vi "Main Abstraction Level 4.vi"() -> ()   [LabVIEW 2019]
doc: "This is one of the levels of abstract design along the timeline leading to the goal of a complete measurement application."
uses:
  messages/MeasureAndLogMessage.lvclass/MeasureAndLogMessage.ctl
  subVIs/Measure and Log Settings.ctl
  subVIs/Simulated Signal Type.ctl
  <extravilib>/ChannelInstances/Stream-str/Read With Abort.vi
  <extravilib>/ChannelInstances/Lossy Stream-a[.](wfm(dbl))/Read With Abort.vi
  <resource>/Channels/Messenger/Read With Abort.vi
  <vilib>/ChannelSupport/Channel Message/Read ID.vi
  <extravilib>/ChannelInstances/Stream-a[.](wfm(dbl))/Endpoint.vi
  <extravilib>/ChannelInstances/Stream-str/EndpointRead.vi
  <extravilib>/ChannelInstances/Lossy Stream-a[.](wfm(dbl))/EndpointRead.vi
  <extravilib>/ChannelInstances/Lossy Stream-a[.](wfm(dbl))/Endpoint.vi
  <extravilib>/ChannelInstances/Stream-str/Endpoint.vi
  messages/MeasureAndLogMessage.lvclass
  e:/builds/penguin/labview/branches/2019/dev/dist/vi.lib/ChannelSupport/Channel Message/Channel Message.lvclass
  <extravilib>/ChannelInstances/Tag-path/Instantiate.vi
  <extravilib>/ChannelInstances/Stream-a[.](wfm(dbl))/Instantiate.vi
  <extravilib>/ChannelInstances/Lossy Stream-a[.](wfm(dbl))/Instantiate.vi
  <extravilib>/ChannelInstances/Lossy Stream-a[.](wfm(dbl))/)Channel.vi
  <resource>/ChannelSupport/_ChannelSupport/WaitIfNeeded.vi
  <extravilib>/ChannelInstances/Stream-str/Instantiate.vi
  <extravilib>/ChannelInstances/Stream-str/)Channel.vi
  <resource>/Channels/Messenger/Instantiate.vi
  <resource>/Channels/Messenger/Endpoint.vi
  <extravilib>/ChannelInstances/Tag-path/Endpoint.vi
  <extravilib>/ChannelInstances/Stream-a[.](wfm(dbl))/)Channel.vi
  <resource>/Channels/Messenger/Messenger.lvlib
  <extravilib>/ChannelInstances/Stream-str.lvlib
  <extravilib>/ChannelInstances/Lossy Stream-a[.](wfm(dbl)).lvlib
  <extravilib>/ChannelInstances/Tag-path.lvlib
  <extravilib>/ChannelInstances/Stream-a[.](wfm(dbl)).lvlib
panel:
  in  "Exit flag":bool
  in  "Record":bool
  in  "Stop":bool
  out "Data":waveform(dbl)[](graph)
  out "Status":string
  in  "Settings":bool
  in  "Start":bool
  in  "Exit":bool
  # "Continuous Measurement Data Logger"
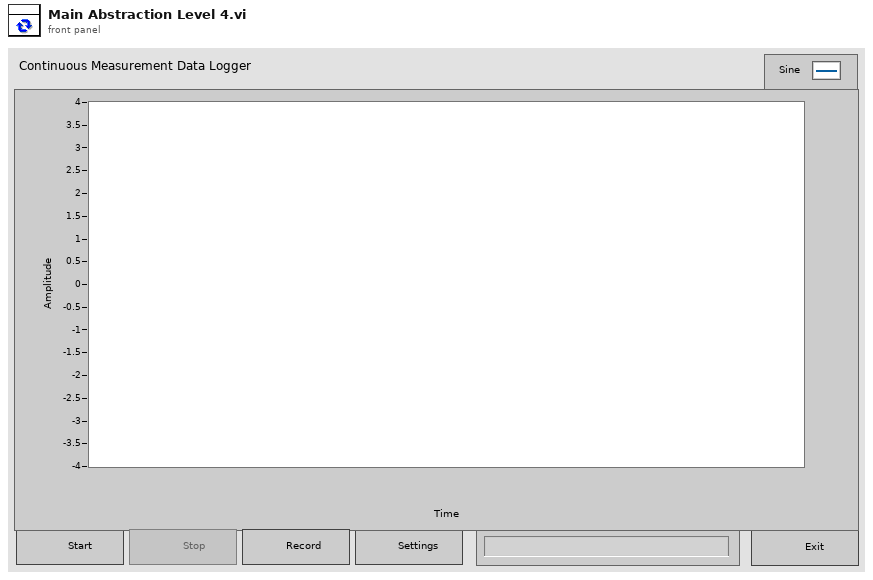
[diagram p1: front panel]
types:
  T1 = typedef "Measure and Log Settings.ctl" = cluster{"sample rate":dbl, "input range":dbl, "logfile path":path, "Simulated Signal":cluster{"signal type":T2, "frequency":dbl, "amplitude":dbl}}
  T2 = typedef "Simulated Signal Type.ctl" = enum16{"Sine Wave", "Square Wave with Noise"}
  T3 = enum8{"Enabled", "Disabled", "Disabled and Grayed Out"}
  T4 = typedef "Messenger.lvlib/))Channel.ctl" = refnum<queue>
  T5 = typedef "Tag-path.lvlib/))Channel.ctl" = refnum<queue>
  T6 = typedef "Stream-a[.](wfm(dbl)).lvlib/)Channel.ctl" = refnum<queue>
  T7 = typedef "Stream-str.lvlib/)Channel.ctl" = refnum<queue>
  T8 = typedef "Lossy Stream-a[.](wfm(dbl)).lvlib/)Channel.ctl" = refnum<queue>
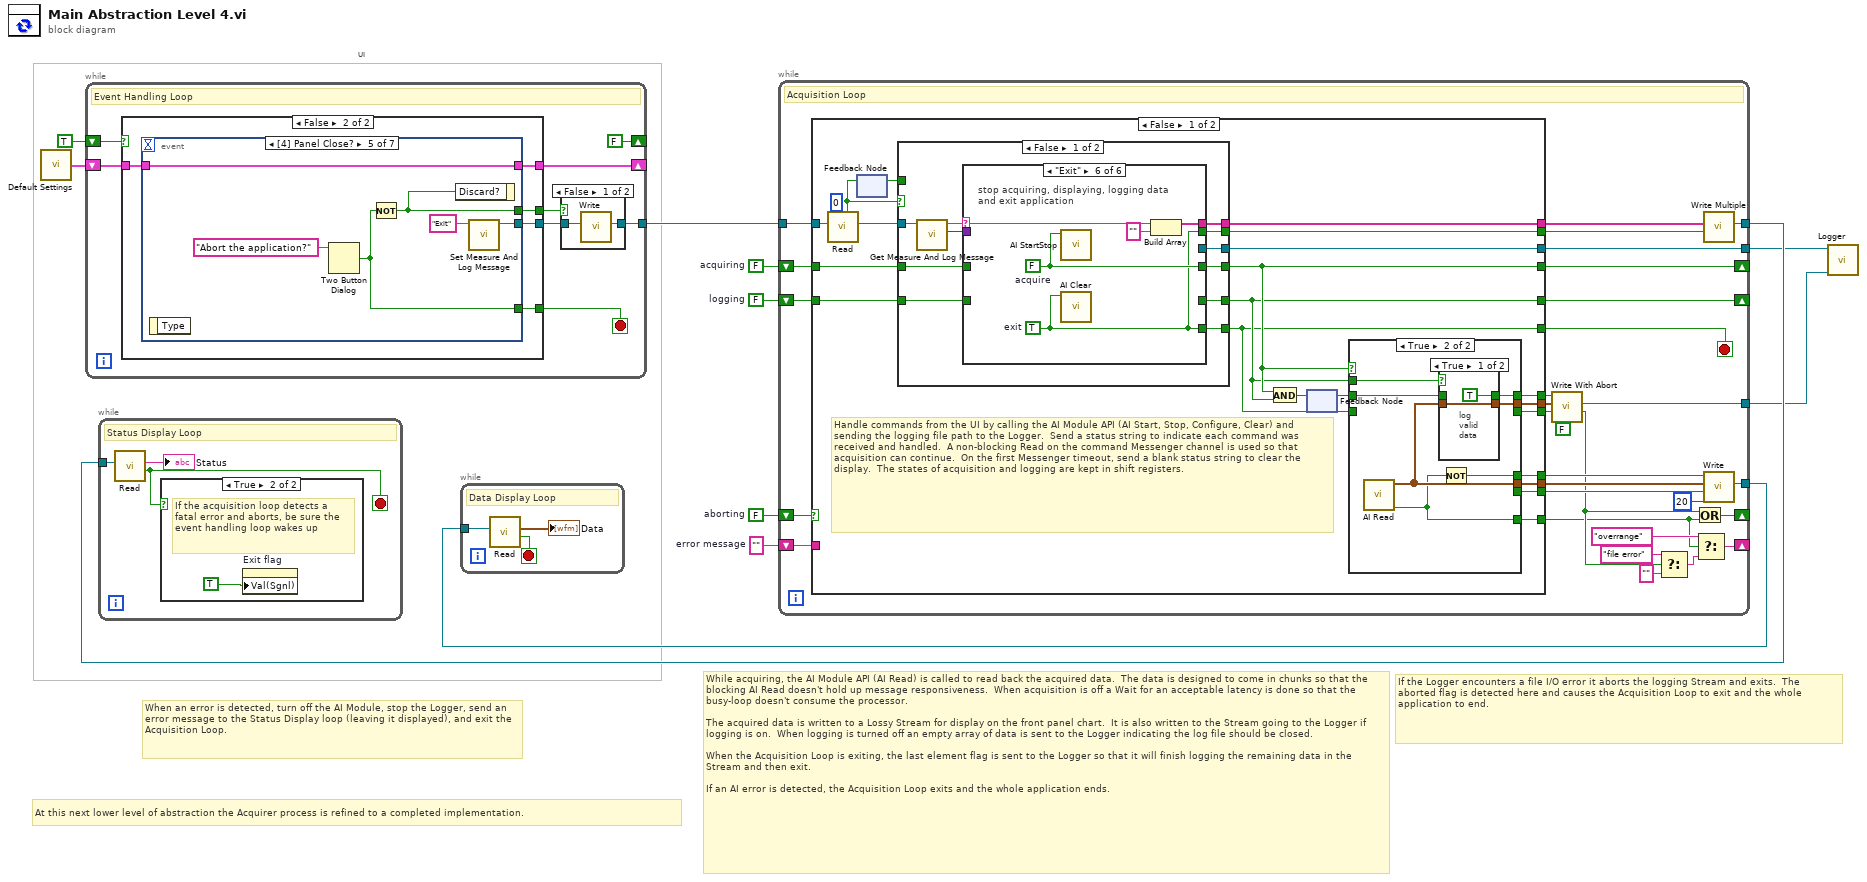
[diagram p0: block diagram]
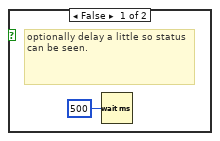
[diagram p2: hidden frame]
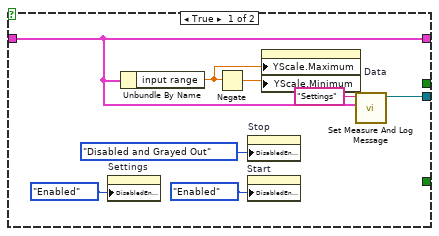
[diagram p3: hidden frame]
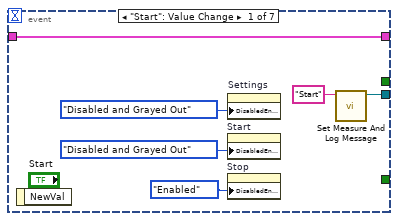
[diagram p4: hidden frame]
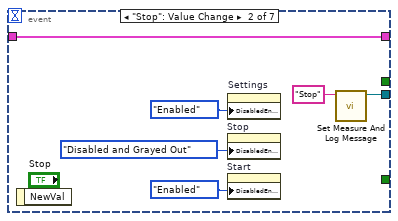
[diagram p5: hidden frame]
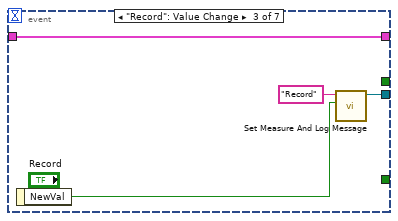
[diagram p6: hidden frame]
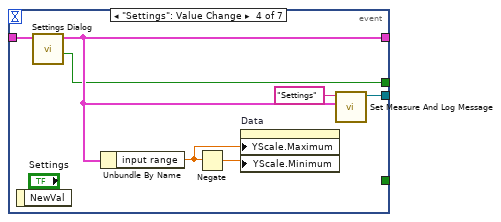
[diagram p7: hidden frame]
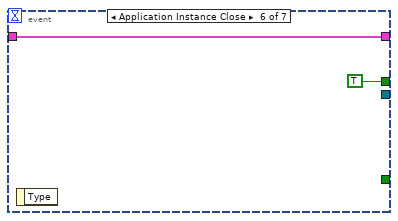
[diagram p8: hidden frame]
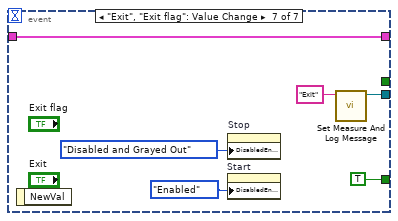
[diagram p9: hidden frame]
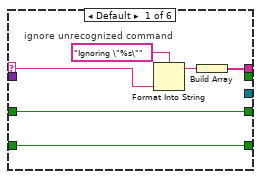
[diagram p11: hidden frame]
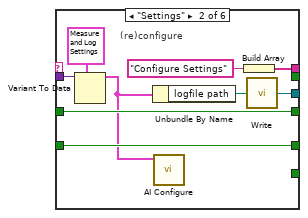
[diagram p12: hidden frame]
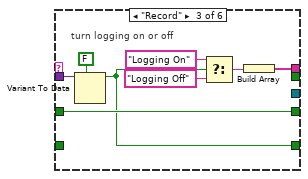
[diagram p13: hidden frame]
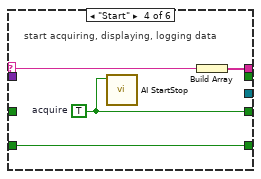
[diagram p14: hidden frame]
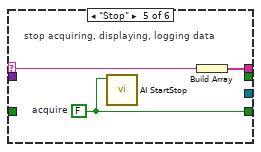
[diagram p15: hidden frame]
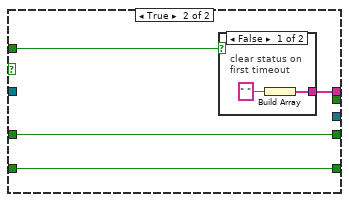
[diagram p16: hidden frame]
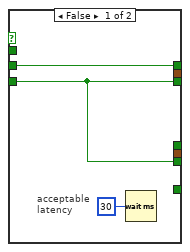
[diagram p18: hidden frame]
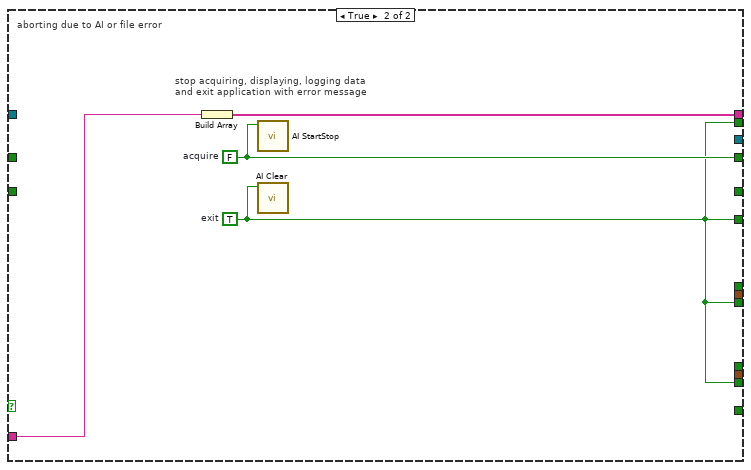
[diagram p20: hidden frame]
diagram:
  w6 = ""  # error message
  w8 = FALSE  # aborting
  w9 = FALSE  # logging
  w10 = FALSE  # acquiring
  # "At this next lower level of abstraction the Acquirer process is refined to a completed implementation."
  # "When an error is detected, turn off the AI Module, stop the Logger, send an error message to the Status Display loop (leaving it displayed), and exit the Acquisition Loop."
  # "If the Logger encounters a file I/O error it aborts the logging Stream and exits.  The aborted flag is detected here and causes the Acquisition Loop to exit and the whole application to end."
  # "While acquiring, the AI Module API (AI Read) is called to read back the acquired data.  The data is designed to come in chunks so that the blocking AI Read doesn't hold up message responsiveness.  When acquisition is off a Wait for an acceptable latency is done so that the busy-loop doesn't consume the processor.\n\nThe acquired data is written to a Lossy Stream for display on the front panel chart.  It is also written to the Stream going to the Logger if logging is on.  When logging is turned off an empty array of data is sent to the Logger indicating the log file should be closed.\n\nWhen the Acquisition Loop is exiting, the last element flag is sent to the Logger so that it will finish logging the remaining data in the Stream and then exit.\n\nIf an AI error is detected, the Acquisition Loop exits and the whole application ends."
  # "UI"
  n1 = call "Default Settings.vi"() -> ("default settings"=w7:T1)
  n2 = while {
    tunnel: [w16] -> w11
    shift-right: [w18] -> _
    shift-left: w7 -> [w17]
    shift-right: [FALSE] -> _
    shift-left: TRUE -> [w12]
    stop <- w19 stop-if-true
    # "Event Handling Loop"
    n3 = case shown="False" w12 {
      tunnel: [_ w32] -> w19
      tunnel: [w26 w31] -> w18
      tunnel: w17 -> [w26 w30]
      tunnel: [w22 w29] -> w15
      tunnel: [_ w28] -> w14
      frame True {
        n4 = property on="Settings" class="Bool"("DisabledEnum"=T3."Enabled" ("Disabled")) -> ()  [unwired: 2 in, 2 out]
        n5 = Unbundle By Name(w26) -> ("input range"=w20:dbl)
        n6 = Negate(x=w20) -> (-x=w21:dbl)
        n7 = property on="Stop" class="Bool"("DisabledEnum"=T3."Disabled and Grayed Out" ("Disabled")) -> ()  [unwired: 2 in, 2 out]
        n8 = property on="Start" class="Bool"("DisabledEnum"=T3."Enabled" ("Disabled")) -> ()  [unwired: 2 in, 2 out]
        n9 = property on="Data" class="WFChart (strict)"("YScale.Maximum"=w20, "YScale.Minimum"=w21) -> ()  [unwired: 2 in, 2 out]
        n10 = call "Set Measure And Log Message.vi"("args"=w26, "command"="Settings") -> ("MyMessage"=w22:refnum<class "MeasureAndLogMessage.lvclass">)  [unwired: 9 in]
      }
      frame False {
        n11 = event shown="[4] Panel Close?" {
          selector: _ -> [_ _ _ _ _ _ _]
          dyn-events: _ -> [_ _ _ _ _ _ _]
          timeout: _ -> [_ _ _ _ _ _ _]
          tunnel: [_ _ _ _ w57 _ TRUE] -> w32
          tunnel: [w34 w40 w46 w54 w60 w63 w65] -> w31
          tunnel: w30 -> [w34 w40 w46 w55 w60 w63 w65]
          tunnel: [w33 w39 w45 w53 w58 _ w64] -> w29
          tunnel: [_ _ _ w51 w56 TRUE ("cancelled") _] -> w28
          event "Start": Value Change {
            n12 = event-data() -> ()  [unwired: 1 in, 1 out]
            n13 = property on="Settings" class="Bool"("DisabledEnum"=T3."Disabled and Grayed Out" ("Disabled")) -> ()  [unwired: 2 in, 2 out]
            n14 = property on="Start" class="Bool"("DisabledEnum"=T3."Disabled and Grayed Out" ("Disabled")) -> ()  [unwired: 2 in, 2 out]
            n15 = property on="Stop" class="Bool"("DisabledEnum"=T3."Enabled" ("Disabled")) -> ()  [unwired: 2 in, 2 out]
            n16 = call "Set Measure And Log Message.vi"("command"="Start") -> ("MyMessage"=w33:refnum<class "MeasureAndLogMessage.lvclass">)  [unwired: 10 in]
          }
          event "Stop": Value Change {
            n17 = event-data() -> ()  [unwired: 1 in, 1 out]
            n18 = property on="Settings" class="Bool"("DisabledEnum"=T3."Enabled" ("Disabled")) -> ()  [unwired: 2 in, 2 out]
            n19 = property on="Stop" class="Bool"("DisabledEnum"=T3."Disabled and Grayed Out" ("Disabled")) -> ()  [unwired: 2 in, 2 out]
            n20 = property on="Start" class="Bool"("DisabledEnum"=T3."Enabled" ("Disabled")) -> ()  [unwired: 2 in, 2 out]
            n21 = call "Set Measure And Log Message.vi"("command"="Stop") -> ("MyMessage"=w39:refnum<class "MeasureAndLogMessage.lvclass">)  [unwired: 10 in]
          }
          event "Record": Value Change {
            n22 = event-data() -> ("NewVal"=w47:bool)  [unwired: 1 in]
            n23 = call "Set Measure And Log Message.vi"("args"=w47, "command"="Record") -> ("MyMessage"=w45:refnum<class "MeasureAndLogMessage.lvclass">)  [unwired: 9 in]
          }
          event "Settings": Value Change {
            n24 = event-data() -> ()  [unwired: 1 in, 1 out]
            n25 = call "Settings Dialog.vi"("settings in"=w55) -> ("cancelled"=w51:bool, "settings out"=w54:T1)  [unwired: 9 in]
            n26 = Unbundle By Name(w54) -> ("input range"=w49:dbl)
            n27 = Negate(x=w49) -> (-x=w50:dbl)
            n28 = property on="Data" class="WFChart (strict)"("YScale.Maximum"=w49, "YScale.Minimum"=w50) -> ()  [unwired: 2 in, 2 out]
            n29 = call "Set Measure And Log Message.vi"("args"=w54, "command"="Settings") -> ("MyMessage"=w53:refnum<class "MeasureAndLogMessage.lvclass">)  [unwired: 9 in]
          }
          event Panel Close? {
            n30 = event-data() -> ()  [unwired: 1 in, 1 out]
            n31 = Two Button Dialog(message="Abort the application?") -> (T button?=w57:bool)  [unwired: 2 in]
            n32 = Not(x=w57) -> (.not. x?=w56:bool)
            n33 = event-data("Discard?"=w56) -> ()  [unwired: 1 in, 1 out]
            n34 = call "Set Measure And Log Message.vi"("command"="Exit") -> ("MyMessage"=w58:refnum<class "MeasureAndLogMessage.lvclass">)  [unwired: 10 in]
          }
          event Application Instance Close {
            n35 = event-data() -> ()  [unwired: 1 in, 1 out]
          }
          event "Exit", "Exit flag": Value Change {
            n36 = event-data() -> ()  [unwired: 1 in, 1 out]
            n37 = property on="Stop" class="Bool"("DisabledEnum"=T3."Disabled and Grayed Out" ("Disabled")) -> ()  [unwired: 2 in, 2 out]
            n38 = property on="Start" class="Bool"("DisabledEnum"=T3."Enabled" ("Disabled")) -> ()  [unwired: 2 in, 2 out]
            n39 = call "Set Measure And Log Message.vi"("command"="Exit") -> ("MyMessage"=w64:refnum<class "MeasureAndLogMessage.lvclass">)  [unwired: 10 in]
          }
        }
      }
    }
    n40 = case shown="False" w14 {
      tunnel: [w71 _] -> w16
      tunnel: w15 -> [w70 _]
      frame False {
        n41 = call <extravilib>:"Write.vi"("element"=w70) -> ("channel"=w71:T4)  [unwired: 8 in, 2 out]
      }
      frame True {
      }
    }
  }
  n42 = while {
    tunnel: w11 -> [w100]
    tunnel: [w92] -> w5
    tunnel: [w89] -> w4
    tunnel: [w85] -> w3
    shift-right: [w97] -> _
    shift-left: w10 -> [w98]
    shift-right: [w96] -> _
    shift-left: w9 -> [w101]
    tunnel: [w99] -> w2
    shift-right: [w84] -> _
    shift-left: w8 -> [w95]
    shift-right: [w75] -> _
    shift-left: w6 -> [w94]
    stop <- w93 stop-if-true
    # "Acquisition Loop"
    n43 = case shown="False" w95 {
      tunnel: w101 -> [w123 _]
      tunnel: w100 -> [w122 _]
      tunnel: [w117 _] -> w99
      tunnel: w98 -> [w116 _]
      tunnel: [w115 w190] -> w97
      tunnel: [w114 _] -> w96
      tunnel: [w111 w189] -> w93
      tunnel: w94 -> [_ w192]
      tunnel: [w109 w189] -> w91
      tunnel: [w110 w191] -> w90
      tunnel: [w107 w189] -> w88
      tunnel: [w108 _] -> w87
      tunnel: [w106 _] -> w86
      tunnel: [w105 _] -> w76
      tunnel: [w104 _] -> w83
      tunnel: [w103 w189] -> w82
      tunnel: [w102 _] -> w81
      frame False {
        # "Handle commands from the UI by calling the AI Module API (AI Start, Stop, Configure, Clear) and sending the logging file path to the Logger.  Send a status string to indicate each command was received and handled.  A non-blocking Read on the command Messenger channel is used so that acquisition can continue.  On the first Messenger timeout, send a blank status string to clear the display.  The states of acquisition and logging are kept in shift registers."
        n44 = call <resource>:"Read.vi"("timeout in ms (-1)"=0, "channel"=w122) -> ("element"=w121:refnum<class "Channel Message.lvclass">, "timed out?"=w119:bool)  [unwired: 7 in, 1 out]
        n45 = feedback #1() -> (w118:bool)  [unwired: 1 in]
        n46 = feedback-in #1(w119) -> ()
        n47 = case shown="False" w119 {
          tunnel: w121 -> [w134 _]
          tunnel: [w131 _] -> w111
          tunnel: [w130 w173] -> w115
          tunnel: w116 -> [w129 w173]
          tunnel: [w128 w172] -> w114
          tunnel: w123 -> [w127 w172]
          tunnel: w118 -> [_ w171]
          tunnel: [w126 _] -> w117
          tunnel: [w125 w170] -> w110
          tunnel: [w124 _] -> w109
          frame False {
            n48 = call "Get Measure And Log Message.vi"("MyMessage"=w134) -> ("args"=w132:variant, "command"=w133:string)  [unwired: 7 in, 2 out]
            n49 = case shown="\"Exit\"" w133 {
              selector: w133 -> [w140 _ _ w160 w164 w169]
              tunnel: w132 -> [_ w147 w156 _ _ _]
              tunnel: [_ _ _ _ _ w165] -> w131
              tunnel: [w138 w149 w157 w158 w162 w166] -> w130
              tunnel: w129 -> [w138 w149 w157 _ _ _]
              tunnel: [w137 w148 w152 w161 _ _] -> w128
              tunnel: w127 -> [w137 w148 _ w161 _ _]
              tunnel: [_ w145 _ _ _ _] -> w126
              tunnel: [w135 w142 w150 w159 w163 w167] -> w125
              tunnel: [_ _ _ _ _ w165] -> w124
              frame Default {
                # "ignore unrecognized command"
                n50 = Format Into String(format string="Ignoring \"%s\"", w140) -> (resulting string=w136:string)  [unwired: 2 in, 1 out]
                n51 = Build Array(w136) -> (w135:string[])
              }
              frame "Settings" {
                # "(re)configure"
                n52 = Variant To Data(type=T1 {"sample rate"=100.0, "input range"=10.0, "logfile path"=path "/Volumes/Bohr/Users/jeffk/Documents/LabVIEW Data/Logged Data.tdms", "Simulated Signal"={"signal type"=enum."Sine Wave", "frequency"=1000.0, "amplitude"=5.0}} ("settings out"), Variant=w147) -> (data=w141:T1)  [unwired: 1 in, 1 out]
                n53 = Unbundle By Name(w141) -> ("logfile path"=w146:path)
                n54 = call "AI Configure.vi"("settings in"=w141) -> ()  [unwired: 11 in]
                n55 = Build Array("Configure Settings" ("element")) -> (w142:string[])
                n56 = call <extravilib>:"Write.vi"("element"=w146) -> ("channel"=w145:T5)  [unwired: 1 out]
              }
              frame "Record" {
                # "turn logging on or off"
                n57 = Variant To Data(type=FALSE, Variant=w156) -> (data=w152:bool)  [unwired: 1 in, 1 out]
                n58 = Select(t="Logging On", s=w152, f="Logging Off") -> (s? t:f=w151:string)
                n59 = Build Array(w151) -> (w150:string[])
              }
              frame "Start" {
                w158 = TRUE  # acquire
                # "start acquiring, displaying, logging data"
                n60 = call "AI StartStop.vi"("acquire"=w158) -> ()  [unwired: 11 in]
                n61 = Build Array(w160) -> (w159:string[])
              }
              frame "Stop" {
                w162 = FALSE  # acquire
                # "stop acquiring, displaying, logging data"
                n62 = call "AI StartStop.vi"("acquire"=w162) -> ()  [unwired: 11 in]
                n63 = Build Array(w164) -> (w163:string[])
              }
              frame "Exit" {
                w166 = FALSE  # acquire
                w165 = TRUE  # exit
                # "stop acquiring, displaying, logging data\nand exit application"
                n64 = call "AI StartStop.vi"("acquire"=w166) -> ()  [unwired: 11 in]
                n65 = call "AI Clear.vi"("clear"=w165) -> ()  [unwired: 11 in]
                n66 = Build Array(w169, "" ("element")) -> (w167:string[])
              }
            }
          }
          frame True {
            n67 = case shown="False" w171 {
              tunnel: [w174 _] -> w170
              frame False {
                # "clear status on\nfirst timeout"
                n68 = Build Array(" " ("string")) -> (w174:string[])
              }
              frame True {
              }
            }
          }
        }
        n69 = And(x=w115, y=w114) -> (x .and. y?=w113:bool)
        n70 = feedback #2() -> (w112:bool)  [unwired: 1 in]
        n71 = feedback-in #2(w113) -> ()
        n72 = case shown="True" w115 {
          tunnel: w114 -> [_ w185]
          tunnel: w112 -> [w178 w184]
          tunnel: w111 -> [w177 _]
          tunnel: [_ w183] -> w108
          tunnel: [w177 _] -> w107
          tunnel: [_ w180] -> w106
          tunnel: [_ w179] -> w105
          tunnel: [w178 w181] -> w104
          tunnel: [w177 _] -> w103
          tunnel: [_ w182] -> w102
          frame False {
            # "acceptable\nlatency"
            n73 = Wait (ms)(milliseconds to wait=u32 30) -> ()  [unwired: 1 out]
          }
          frame True {
            n74 = call "AI Read.vi"() -> ("error"=w179:bool, "waveforms"=w180:waveform(dbl)[])  [unwired: 10 in]
            n75 = case shown="True" w185 {
              tunnel: w180 -> [w187 _]
              tunnel: w184 -> [_ w188]
              tunnel: [w187 _] -> w182
              tunnel: [TRUE w188] -> w181
              frame True {
                # "log \nvalid\ndata"
              }
              frame False {
              }
            }
            n76 = Not(x=w179) -> (.not. x?=w183:bool)
          }
        }
      }
      frame True {
        w190 = FALSE  # acquire
        w189 = TRUE  # exit
        # "aborting due to AI or file error"
        # "stop acquiring, displaying, logging data\nand exit application with error message"
        n77 = Build Array(w192) -> (w191:string[])
        n78 = call "AI StartStop.vi"("acquire"=w190) -> ()  [unwired: 11 in]
        n79 = call "AI Clear.vi"("clear"=w189) -> ()  [unwired: 11 in]
      }
    }
    n80 = call <extravilib>:"Write With Abort.vi"("abort"=FALSE, "last element? (F)"=w82, "element"=w81, "element valid? (T)"=w83) -> ("aborted?"=w79:bool, "channel"=w85:T6)  [unwired: 4 in, 2 out]
    n81 = Select(t="file error", s=w79, f="") -> (s? t:f=w74:string)
    n82 = Or(x=w79, y=w76) -> (x .or. y?=w84:bool)
    n83 = Select(t="overrange", s=w76, f=w74) -> (s? t:f=w75:string)
    n84 = call <extravilib>:"Write Multiple.vi"("last element? (F)"=w91, "elements"=w90) -> ("channel"=w92:T7)  [unwired: 6 in, 3 out]
    n85 = call <extravilib>:"Write.vi"("size (1)"=20, "last element? (F)"=w88, "element"=w86, "element valid? (T)"=w87) -> ("channel"=w89:T8)  [unwired: 5 in, 2 out]
  }
  n86 = while {
    tunnel: w5 -> [w195]
    stop <- w193 stop-if-true
    # "Status Display Loop"
    n87 = call <resource>:"Read.vi"("channel"=w195) -> ("last element?"=w193:bool, "element"=→"Status":string)  [unwired: 6 in, 3 out]
    n88 = case shown="True" w193 {
      frame False {
        # "optionally delay a little so status can be seen."
        n89 = Wait (ms)(milliseconds to wait=u32 500) -> ()  [unwired: 1 out]
      }
      frame True {
        # "If the acquisition loop detects a fatal error and aborts, be sure the event handling loop wakes up"
        n90 = property on="Exit flag" class="Bool (strict)"("Val(Sgnl)"=TRUE) -> ()  [unwired: 2 in, 2 out]
      }
    }
  }
  n91 = while {
    tunnel: w4 -> [w198]
    stop <- w200 stop-if-true
    # "Data Display Loop"
    n92 = call <resource>:"Read.vi"("channel"=w198) -> ("last element?"=w200:bool, "element"=→"Data":waveform(dbl)[])  [unwired: 5 in, 4 out]
  }
  n93 = call "Logger.vi"("wfm data stream"=w3, "file path tag"=w2) -> ()  [unwired: 9 in, 1 out]
